vi "_getTempValueOfAllPortsRead_EEPROM_VNA_wmg.vi"(0 "AA or AB?":bool=TRUE, 5 "portNum":i32, 7 "ref_W&R_ports":refnum<vi>[](array[refnum]), 9 "AA or AB inf":i32[](array[numeric]), 11 "info_read":string[][](array[string])) -> (4 "temp port0":string[][](array[string]), 6 "temp port1":string[][](array[string]), 10 "temp port2":string[][](array[string]), 14 "temp port4":string[][](array[string]), 15 "temp port3":string[][](array[string]))   [LabVIEW 2011]
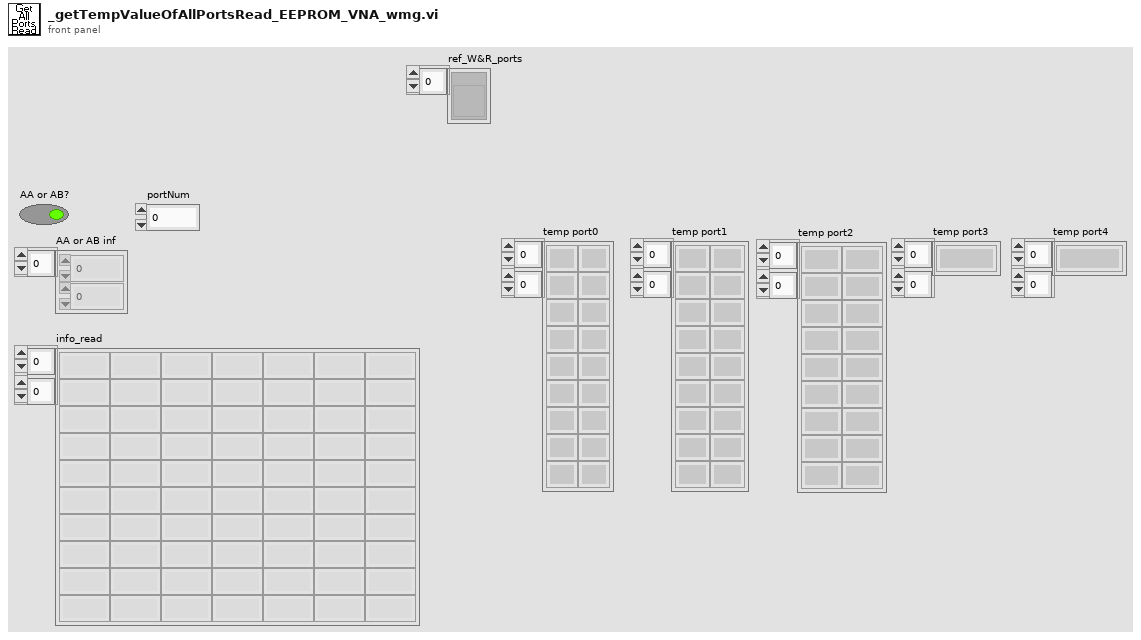
[diagram p1: front panel]
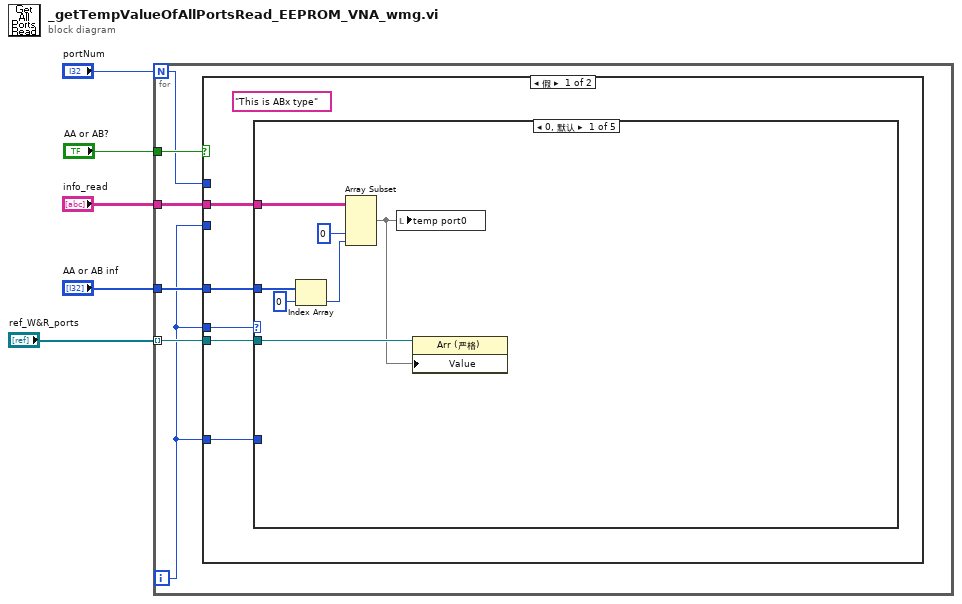
[diagram p0: block diagram]
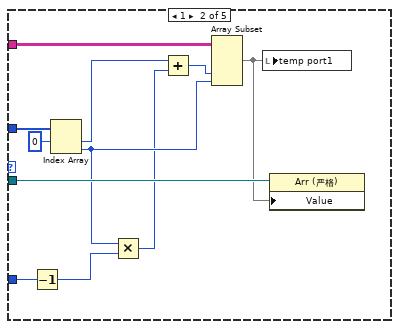
[diagram p2: hidden frame]
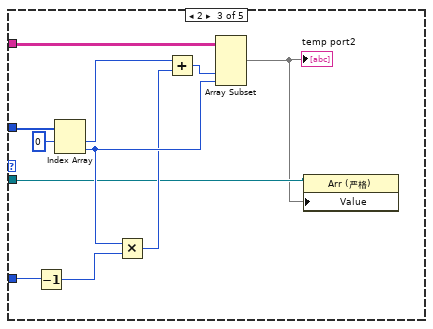
[diagram p3: hidden frame]
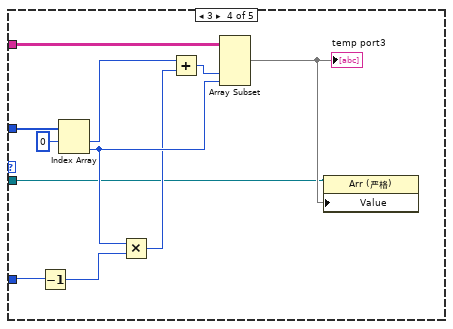
[diagram p4: hidden frame]
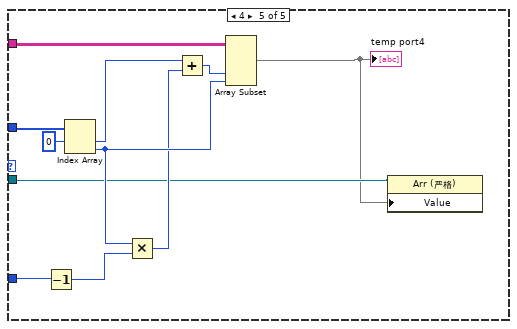
[diagram p5: hidden frame]
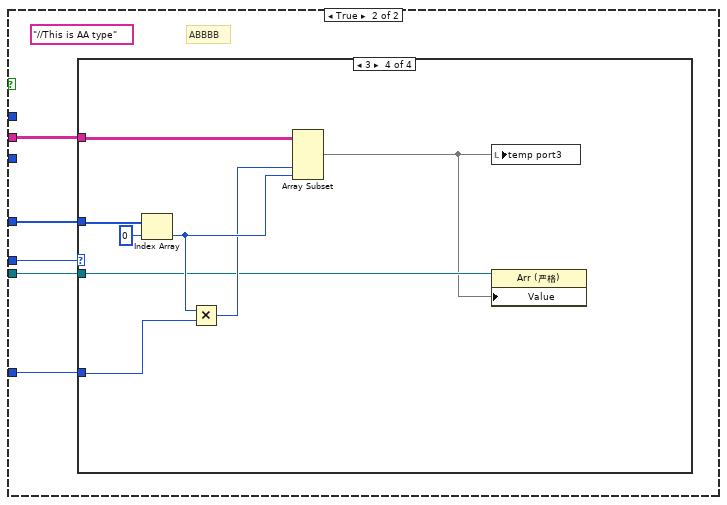
[diagram p6: hidden frame]
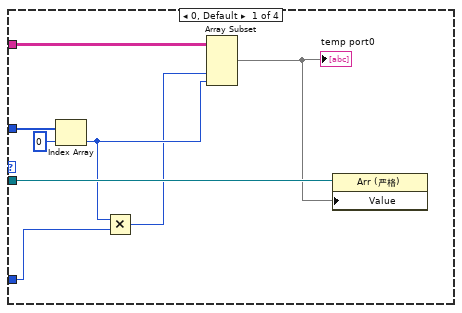
[diagram p7: hidden frame]
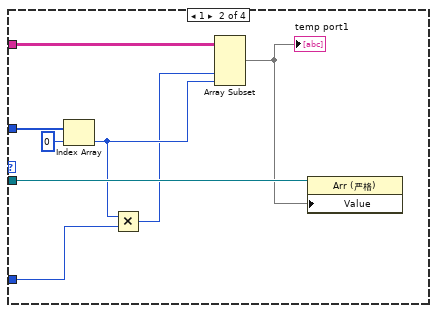
[diagram p8: hidden frame]
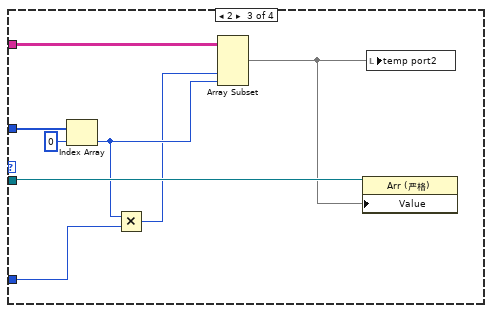
[diagram p9: hidden frame]
diagram:
  n1 = for {
    N: "portNum" -> [w9]
    tunnel: "AA or AB?" -> [w11]
    tunnel: "info_read" -> [w10]
    tunnel: "AA or AB inf" -> [w8]
    tunnel: "ref_W&R_ports" -> [w7] mode=indexing
    i -> [w6]
    n2 = case shown="假" w11 {
      tunnel: w10 -> [w15 w71]
      tunnel: w6 -> [_ _]
      tunnel: w6 -> [w16 w72]
      tunnel: w9 -> [_ _]
      tunnel: w8 -> [w14 w69]
      tunnel: w7 -> [w13 w70]
      tunnel: w6 -> [w12 w68]
      frame False {
        (unwired) "This is ABx type"
        n3 = case shown="0, 默认" w16 {
          tunnel: w15 -> [w21 w32 w40 w51 w62]
          tunnel: w14 -> [w23 w34 w39 w50 w61]
          tunnel: w13 -> [w18 w31 w38 w47 w59]
          tunnel: w12 -> [_ w29 w37 w49 w60]
          frame 0, Default {
            n4 = Index Array(array=w23, index=0 ("索引")) -> (element=w19:i32)
            n5 = Array Subset(array=w21, index (col)=0 ("索引"), length (col)=w19) -> (w17:string[][])  [unwired: 2 in]
            n6 = local write "temp port0"(w17) -> ()
            n7 = property class="Arr (严格)"(reference=w18, "Value"=w17) -> ()  [unwired: 1 in, 2 out]
          }
          frame 1 {
            n8 = Decrement(x=w29) -> (x-1=w28:i32)
            n9 = Index Array(array=w34, index #1=0 ("索引")) -> (element #1=w26:i32, element #2=w27:i32)  [unwired: 1 in]
            n10 = Multiply(x=w27, y=w28) -> (x*y=w25:i32)
            n11 = Add(x=w26, y=w25) -> (x+y=w24:i32)
            n12 = Array Subset(array=w32, index (col)=w24, length (col)=w27) -> (w30:string[][])  [unwired: 2 in]
            n13 = local write "temp port1"(w30) -> ()
            n14 = property class="Arr (严格)"(reference=w31, "Value"=w30) -> ()  [unwired: 1 in, 2 out]
          }
          frame 2 {
            n15 = Decrement(x=w37) -> (x-1=w44:i32)
            n16 = Index Array(array=w39, index #1=0 ("索引")) -> (element #1=w42:i32, element #2=w43:i32)  [unwired: 1 in]
            n17 = Multiply(x=w43, y=w44) -> (x*y=w41:i32)
            n18 = Add(x=w42, y=w41) -> (x+y=w35:i32)
            n19 = Array Subset(array=w40, index (col)=w35, length (col)=w43) -> (w36:string[][])  [unwired: 2 in]
            "temp port2" <- w36
            n20 = property class="Arr (严格)"(reference=w38, "Value"=w36) -> ()  [unwired: 1 in, 2 out]
          }
          frame 3 {
            n21 = Decrement(x=w49) -> (x-1=w55:i32)
            n22 = Index Array(array=w50, index #1=0 ("索引")) -> (element #1=w53:i32, element #2=w54:i32)  [unwired: 1 in]
            n23 = Multiply(x=w54, y=w55) -> (x*y=w52:i32)
            n24 = Add(x=w53, y=w52) -> (x+y=w46:i32)
            n25 = Array Subset(array=w51, index (col)=w46, length (col)=w54) -> (w48:string[][])  [unwired: 2 in]
            "temp port3" <- w48
            n26 = property class="Arr (严格)"(reference=w47, "Value"=w48) -> ()  [unwired: 1 in, 2 out]
          }
          frame 4 {
            n27 = Decrement(x=w60) -> (x-1=w66:i32)
            n28 = Index Array(array=w61, index #1=0 ("索引")) -> (element #1=w64:i32, element #2=w65:i32)  [unwired: 1 in]
            n29 = Multiply(x=w65, y=w66) -> (x*y=w63:i32)
            n30 = Add(x=w64, y=w63) -> (x+y=w57:i32)
            n31 = Array Subset(array=w62, index (col)=w57, length (col)=w65) -> (w58:string[][])  [unwired: 2 in]
            "temp port4" <- w58
            n32 = property class="Arr (严格)"(reference=w59, "Value"=w58) -> ()  [unwired: 1 in, 2 out]
          }
        }
      }
      frame True {
        (unwired) "//This is AA type"
        # "ABBBB"
        n33 = case shown="3" w72 {
          tunnel: w71 -> [w78 w86 w92 w101]
          tunnel: w70 -> [w80 w88 w96 w98]
          tunnel: w69 -> [w77 w85 w91 w100]
          tunnel: w68 -> [w74 w82 w90 w99]
          frame 0, Default {
            n34 = Index Array(array=w77, index=0 ("索引")) -> (element=w75:i32)
            n35 = Multiply(x=w75, y=w74) -> (x*y=w73:i32)
            n36 = Array Subset(array=w78, index (col)=w73, length (col)=w75) -> (w76:string[][])  [unwired: 2 in]
            "temp port0" <- w76
            n37 = property class="Arr (严格)"(reference=w80, "Value"=w76) -> ()  [unwired: 1 in, 2 out]
          }
          frame 1 {
            n38 = Index Array(array=w85, index=0 ("索引")) -> (element=w83:i32)
            n39 = Multiply(x=w83, y=w82) -> (x*y=w81:i32)
            n40 = Array Subset(array=w86, index (col)=w81, length (col)=w83) -> (w84:string[][])  [unwired: 2 in]
            "temp port1" <- w84
            n41 = property class="Arr (严格)"(reference=w88, "Value"=w84) -> ()  [unwired: 1 in, 2 out]
          }
          frame 2 {
            n42 = Index Array(array=w91, index=0 ("索引")) -> (element=w94:i32)
            n43 = Multiply(x=w94, y=w90) -> (x*y=w93:i32)
            n44 = Array Subset(array=w92, index (col)=w93, length (col)=w94) -> (w89:string[][])  [unwired: 2 in]
            n45 = property class="Arr (严格)"(reference=w96, "Value"=w89) -> ()  [unwired: 1 in, 2 out]
            n46 = local write "temp port2"(w89) -> ()
          }
          frame 3 {
            n47 = Index Array(array=w100, index=0 ("索引")) -> (element=w103:i32)
            n48 = Multiply(x=w103, y=w99) -> (x*y=w102:i32)
            n49 = Array Subset(array=w101, index (col)=w102, length (col)=w103) -> (w97:string[][])  [unwired: 2 in]
            n50 = local write "temp port3"(w97) -> ()
            n51 = property class="Arr (严格)"(reference=w98, "Value"=w97) -> ()  [unwired: 1 in, 2 out]
          }
        }
      }
    }
  }
